vi "SG_WriteSpectrum.vi"(8 "error in":errorcluster, 11 "Spectrum":waveform(dbl)[](array[waveform])) -> (0 "error out":errorcluster)   [LabVIEW 2016]
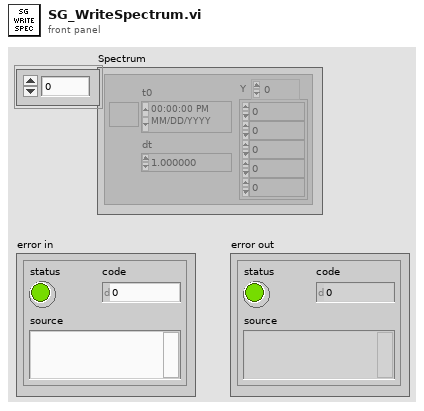
[diagram p1: front panel]
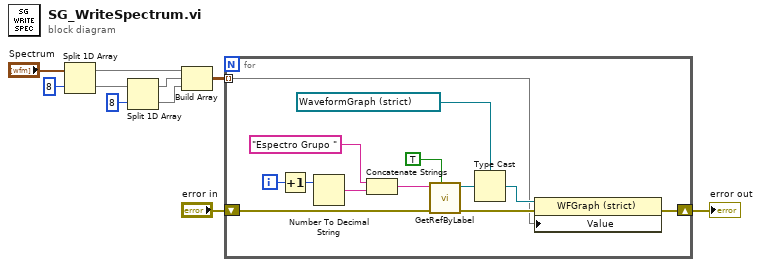
[diagram p0: block diagram]
diagram:
  n1 = Split 1D Array(array="Spectrum", index=8) -> (first subarray=w6:waveform(dbl)[], second subarray=w5:waveform(dbl)[])
  n2 = Split 1D Array(array=w5, index=8) -> (first subarray=w7:waveform(dbl)[], second subarray=w8:waveform(dbl)[])
  n3 = Build Array(w6, w7, w8) -> (w1:waveform(dbl)[][])
  n4 = for {
    tunnel: w1 -> [w12] mode=indexing
    shift-right: [w21] -> w10
    shift-left: "error in" -> [w19]
    i -> [w17]
    n5 = Increment(x=w17) -> (x+1=w13:i32)
    n6 = Number To Decimal String(number=w13) -> (decimal integer string=w16:string)  [unwired: 1 in]
    n7 = Concatenate Strings("Espectro Grupo " ("Label"), w16) -> (w14:string)
    n8 = call "GetRefByLabel.vi"("InsideTab"=TRUE, "error in"=w19, "Label"=w14) -> ("error out"=w18:errorcluster, "Ctl Refnum"=w22:refnum<vi>)  [unwired: 6 in, 1 out]
    n9 = Type Cast(type=refnum<vi> refnum ("Espectro Grupo 1"), x=w22) -> (*(type *) &x=w20:refnum<vi>)
    n10 = property class="WFGraph (strict)"(reference=w20, error in=w18, "Value"=w12) -> (error out=w21:errorcluster)  [unwired: 1 out]
  }
  "error out" <- w10
